vi "Configure Display Window.vi"(7 "Mode (0: Create)":u16(ring) items=["Create", "Delete"], 8 "Error In (no error)":errorcluster, 9 "Display Title String (MY_DISPLAY)":string="MY_DISPLAY", 10 "Display Window (1)":i32=1, 11 "VISA Resource Name":refnum<visa-resource-name>) -> (0 "Error Out":errorcluster, 3 "VISA Resource Name Out":refnum<visa-resource-name>)   [LabVIEW 2018, in "Agilent PNA Series.lvlib"]
doc: "This VI creates or deletes a display window."
uses:
  Agilent PNA Series.lvlib
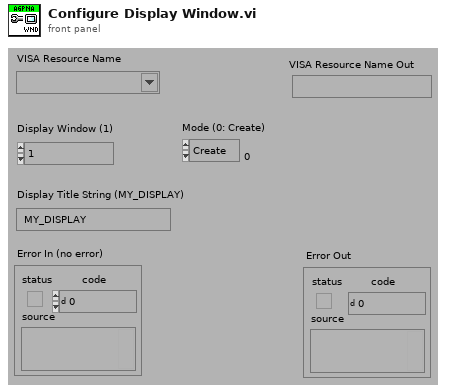
[diagram p1: front panel]
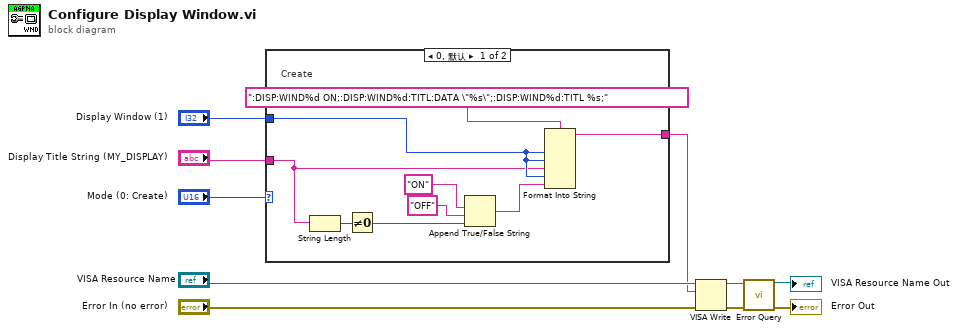
[diagram p0: block diagram]
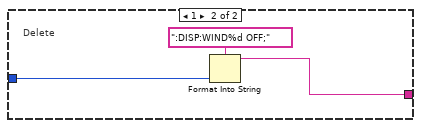
[diagram p2: hidden frame]
diagram:
  n1 = case shown="0, 默认" "Mode (0: Create)" {
    tunnel: [w19 w20] -> w5
    tunnel: "Display Window (1)" -> [w13 w21]
    tunnel: "Display Title String (MY_DISPLAY)" -> [w11 _]
    frame 0, Default {
      # "Create"
      n2 = String Length(string=w11) -> (length=w17:i32)
      n3 = Not Equal To 0?(x=w17) -> (x != 0?=w16:bool)
      n4 = Append True/False String(1:w16, 2:"OFF" ("false string"), 3:"ON" ("true string")) -> (0:w12:string)  [unwired: 1 in]
      n5 = Format Into String(format string=":DISP:WIND%d ON;:DISP:WIND%d:TITL:DATA \"%s\";:DISP:WIND%d:TITL %s;", w13, w13, w11, w13, w12) -> (resulting string=w19:string)  [unwired: 2 in, 1 out]
    }
    frame 1 {
      # "Delete"
      n6 = Format Into String(format string=":DISP:WIND%d OFF;", w21) -> (resulting string=w20:string)  [unwired: 2 in, 1 out]
    }
  }
  n7 = VISA Write(VISA resource name="VISA Resource Name", write buffer=w5, error in (no error)="Error In (no error)") -> (VISA resource name out=w4:refnum<visa-resource-name>, error out=w3:errorcluster)  [unwired: 1 out]
  n8 = call "Error Query.vi"("VISA Resource Name"=w4, "error in (no error)"=w3) -> ("VISA Resource Name Out"=→"VISA Resource Name Out":refnum<visa-resource-name>, "error out"=→"Error Out":errorcluster)  [unwired: 10 in, 2 out]
